vi "Load Settings from DB.vi"(8 "error in":errorcluster) -> (0 "error out":errorcluster, 3 "Dashboard Data (out)":T1={"Drive PID - Low"={"D"=0.0, "F"=0.0, "RR"=0.0, "IZ"=0.0, "P"=0.0, "I"=0.0}, "Drive PID - High"={"D"=0.0, "F"=0.0, "RR"=0.0, "IZ"=0.0, "P"=0.0, "I"=0.0}, "Vision Settings"={"LED Color"={"Hue"={107.81818389892578, 139.81818389892578}, "Sat"={176.07142857142858, 255.0}, "Val"={40.53571428571429, 255.0}}, "Vision Line"=0.0, "Vision Bottom Clip"=0.0}, "Robot Name"="", "Winch Out"=0.0, "Winch In"=0.0, "Shooter Settings"={"Shooter PID"={"D"=0.0, "F"=0.0, "RR"=0.0, "IZ"=0.0, "P"=0.0, "I"=0.0}, "Instake Belt PID"={"D"=0.0, "F"=0.0, "RR"=0.0, "IZ"=0.0, "P"=0.0, "I"=0.0}, "Shooter Wheel RPM"=0.0, "Instake Belt RPM"=0.0, "Grinder Power"=0.0, "Ramp Up Speed"=0.0}, "Auto Start"=enum."Left"} {"Vision Settings"."LED Color"."Hue" scale=0.0..255.0 scale format="%#_3g"})   [LabVIEW 2016]
uses:
  Dashboard Data.ctl
  PID Settings.ctl
  Vision Data.ctl
  Shooter Settings.ctl
  AutoPositions Type Def.ctl
  Load Save Info.ctl
  <vilib>/Utility/config.llb/Config Data RefNum.ctl
  <vilib>/Utility/config.llb/NI_LVConfig.lvlib
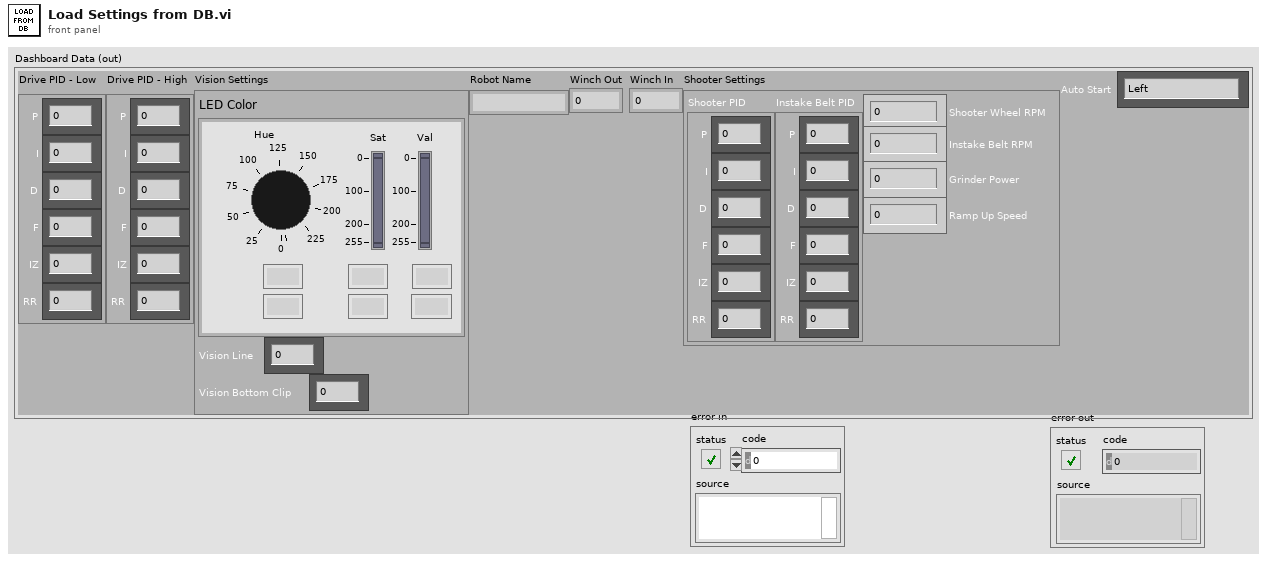
[diagram p1: front panel]
types:
  T1 = typedef "Dashboard Data.ctl" = cluster{"Drive PID - Low":T2, "Drive PID - High":T2, "Vision Settings":T3, "Robot Name":string, "Winch Out":dbl, "Winch In":dbl, "Shooter Settings":T4, "Auto Start":T5}
  T2 = typedef "PID Settings.ctl" = cluster{"D":dbl, "F":dbl, "RR":dbl, "IZ":dbl, "P":dbl, "I":dbl}
  T3 = typedef "Vision Data.ctl" = cluster{"LED Color":cluster{"Hue":cluster{dbl, dbl}, "Sat":cluster{dbl, dbl}, "Val":cluster{dbl, dbl}}, "Vision Line":dbl, "Vision Bottom Clip":dbl}
  T4 = typedef "Shooter Settings.ctl" = cluster{"Shooter PID":T2, "Instake Belt PID":T2, "Shooter Wheel RPM":dbl, "Instake Belt RPM":dbl, "Grinder Power":dbl, "Ramp Up Speed":dbl}
  T5 = typedef "AutoPositions Type Def.ctl" = enum16{"Left", "Middle", "Right"}
  T6 = typedef "Load Save Info.ctl" = cluster{"Load?":bool, "Dashboard?":bool, "save file":T7, "File?":bool}
  T7 = typedef "NI_LVConfig.lvlib/Config Data RefNum.ctl" = refnum<k1>
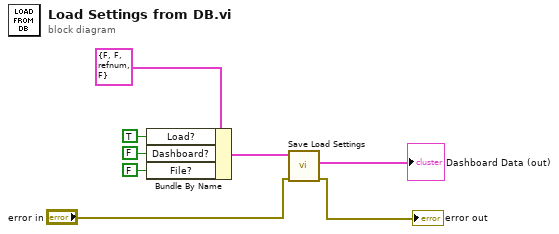
[diagram p0: block diagram]
diagram:
  n1 = Bundle By Name(cluster=T6 {"Load?"=FALSE, "Dashboard?"=FALSE, "save file"=refnum, "File?"=FALSE} ("Save Load Info"), "Load?"=TRUE, "Dashboard?"=FALSE, "File?"=FALSE) -> (w7:T6)
  n2 = call "Save Load Settings.vi"("error in"="error in", "Save Load Info"=w7) -> ("error out"=→"error out":errorcluster, "Dashboard Data (out)"=→"Dashboard Data (out)":T1)  [unwired: 7 in, 1 out]
